vi "Tree Interaction.vi"(10 "Tree Value Changed?":bool, 11 "Settings UI in":refnum<class "Settings UI.lvclass">) -> (3 "Settings UI out":refnum<class "Settings UI.lvclass">)   [LabVIEW 2020, in "Output Sequencer.lvlib" / "Settings UI.lvclass"]
uses:
  Settings UI.lvclass
  Settings UI.lvclass/Settings UI.ctl
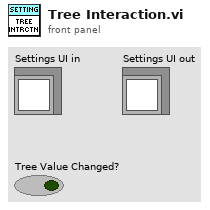
[diagram p1: front panel]
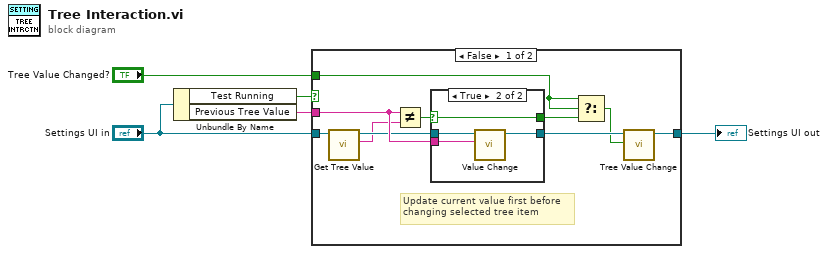
[diagram p0: block diagram]
diagram:
  n1 = Unbundle By Name("Settings UI in") -> ("Test Running"=w4:bool, "Previous Tree Value"=w1:string)
  n2 = case shown="False" w4 {
    tunnel: w1 -> [w15 _]
    tunnel: "Settings UI in" -> [w9 w22]
    tunnel: [w7 w22] -> w3
    tunnel: "Tree Value Changed?" -> [w6 _]
    frame False {
      # "Update current value first before\nchanging selected tree item"
      n3 = call "Get Tree Value.vi"("UI Data in"=w9) -> ("Value"=w12:string, "UI Data out"=w14:refnum<class "Settings UI.lvclass">)  [unwired: 9 in]
      n4 = Not Equal?(x=w15, y=w12) -> (x != y?=w13:bool)
      n5 = case shown="True" w13 {
        selector: w13 -> [w17 w21]
        tunnel: w14 -> [w16 w20]
        tunnel: w15 -> [_ w18]
        tunnel: [w17 w21] -> w11
        tunnel: [w16 w19] -> w10
        frame False {
        }
        frame True {
          n6 = call "Value Change.vi"("Tree Tag"=w18, "UI Data In"=w20) -> ("UI Data Out"=w19:refnum<class "Settings UI.lvclass">)  [unwired: 9 in]
        }
      }
      n7 = Select(t=w6, s=w6, f=w11) -> (s? t:f=w8:bool)
      n8 = call "Tree Value Change.vi"("Selection Changed?"=w8, "UI Data in"=w10) -> ("UI Data out"=w7:refnum<class "Settings UI.lvclass">)  [unwired: 9 in]
    }
    frame True {
    }
  }
  "Settings UI out" <- w3
